vi "advent_2.vi"() -> ()   [LabVIEW 2021]
uses:
  <vilib>/Utility/file.llb/Read Delimited Spreadsheet (string).vi
panel:
  out "old depth equals aim":bool
  out "Horizontals equal?":bool
  out "Aim":i32
  out "horizontal * Depth 2":i32
  out "horizontal 2":i32
  out "Depth 2":i32
  out "min value":i32
  out "max value":i32
  out "size(s)":i32
  out "Depth":i32
  out "horizontal":i32
  out "horizontal * Depth":i32
  out "both same size":bool
  out "all rows":string[][](array[string])
  # "900"
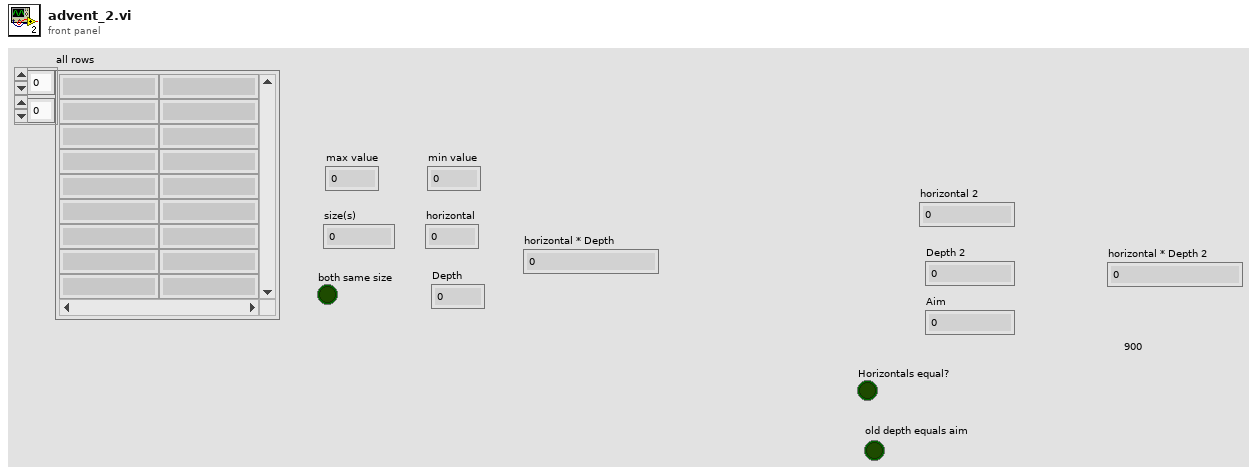
[diagram p1: front panel]
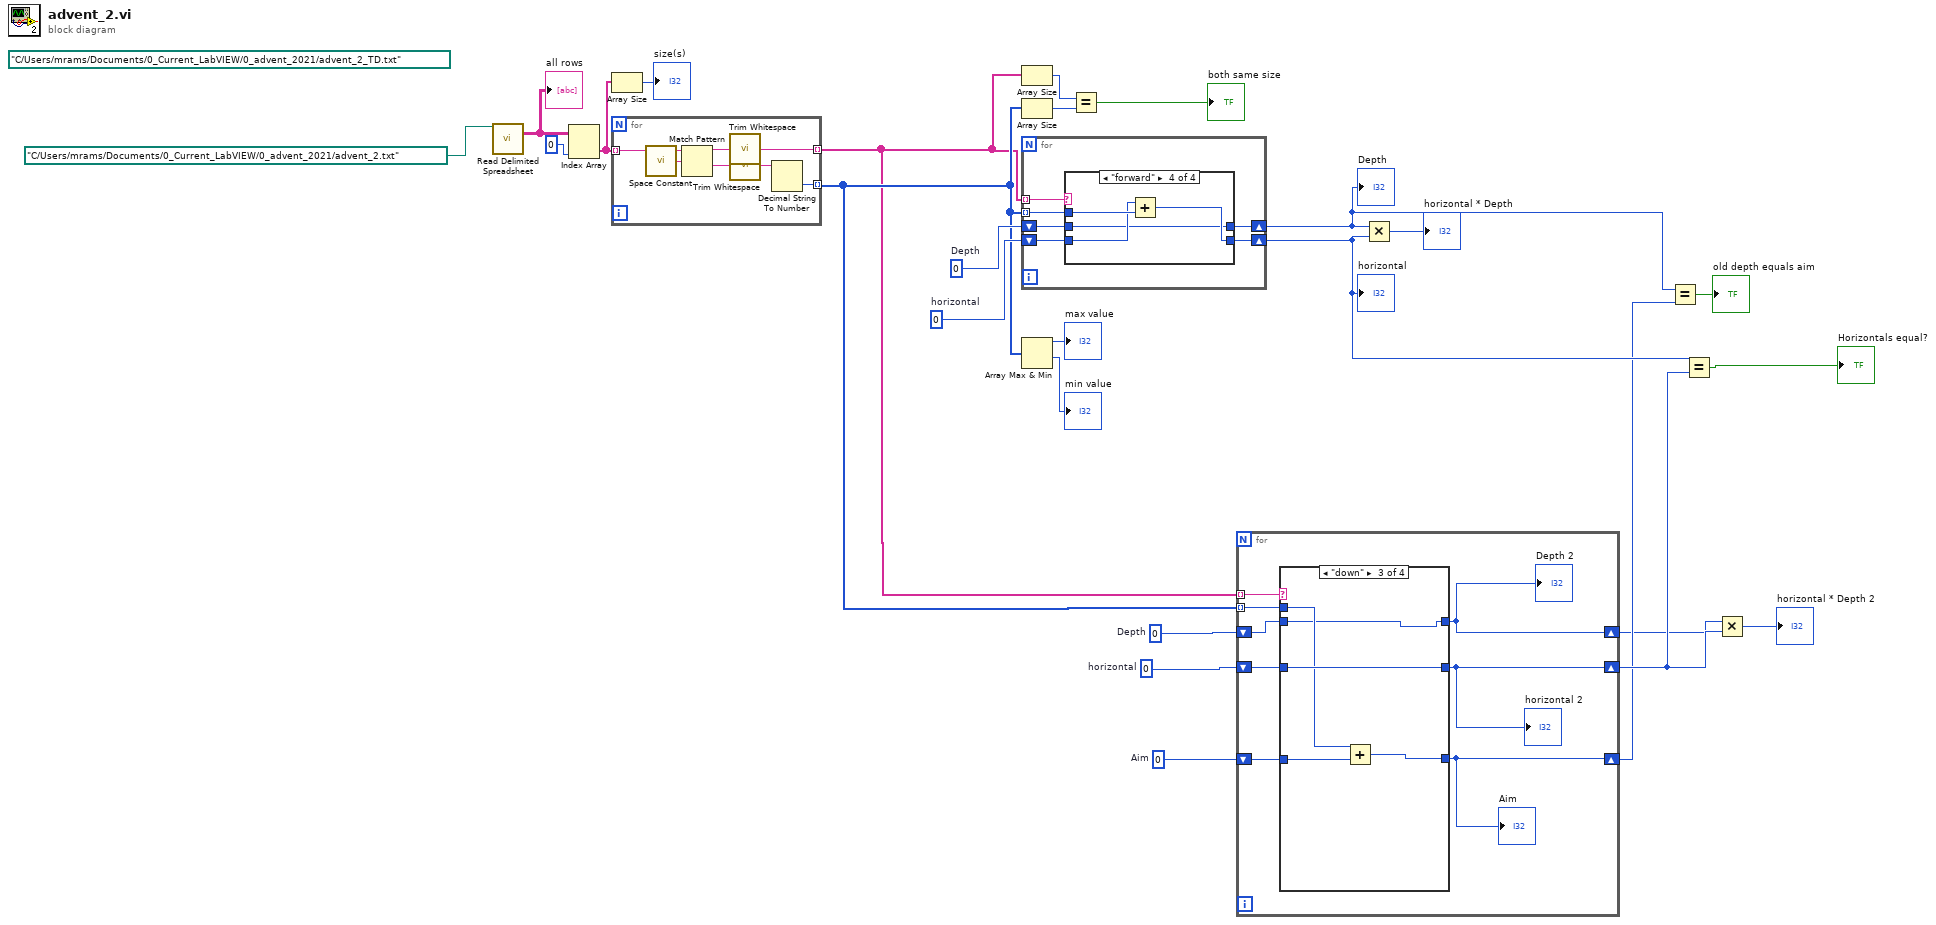
[diagram p0: block diagram]
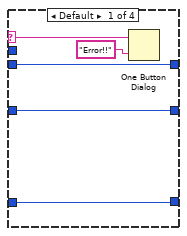
[diagram p2: hidden frame]
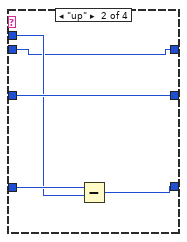
[diagram p3: hidden frame]
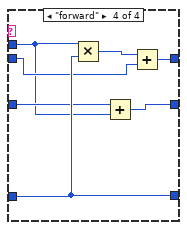
[diagram p4: hidden frame]
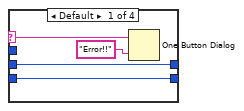
[diagram p5: hidden frame]
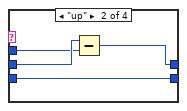
[diagram p6: hidden frame]
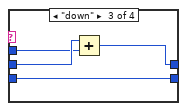
[diagram p7: hidden frame]
diagram:
  (unwired) path "C:/Users/mrams/Documents/0_Current_LabVIEW/0_advent_2021/advent_2_TD.txt" ("file path (dialog if empty)")
  w10 = 0  # Aim
  w12 = 0  # Depth
  w13 = 0  # horizontal
  w21 = 0  # Depth
  w20 = 0  # horizontal
  n1 = call-poly <vilib>:"Read Delimited Spreadsheet.vi"("file path (dialog if empty)"=path "C:/Users/mrams/Documents/0_Current_LabVIEW/0_advent_2021/advent_2.txt") -> ("all rows"=w25:string[][])  [unwired: 9 in, 5 out]
  "all rows" <- w25
  n2 = Index Array(array=w25, index (col)=0 ("disabled index (col)")) -> (element=w18:string[])  [unwired: 1 in]
  n3 = Array Size(array=w18) -> (size(s)=→"size(s)":i32)
  n4 = for {
    tunnel: w18 -> [w32] mode=indexing
    tunnel: [w28] -> w3 mode=indexing
    tunnel: [w29] -> w11 mode=indexing
    n5 = call <vilib>:"Space Constant.vi"() -> ("String"=w33:string)
    n6 = Match Pattern(string=w32, regular expression=w33) -> (before substring=w31:string, after substring=w30:string)  [unwired: 1 in, 2 out]
    n7 = call <vilib>:"Trim Whitespace.vi"("string"=w31) -> ("trimmed string"=w28:string)  [unwired: 1 in]
    n8 = call <vilib>:"Trim Whitespace.vi"("string"=w30) -> ("trimmed string"=w27:string)  [unwired: 1 in]
    n9 = Decimal String To Number(string=w27) -> (number=w29:i32)  [unwired: 2 in, 1 out]
  }
  n10 = Array Size(array=w3) -> (size(s)=w24:i32)
  n11 = Array Size(array=w11) -> (size(s)=w23:i32)
  n12 = for {
    tunnel: w3 -> [w39] mode=indexing
    tunnel: w11 -> [w37] mode=indexing
    shift-right: [w35] -> w5
    shift-left: w21 -> [w38]
    shift-right: [w34] -> w9
    shift-left: w20 -> [w36]
    n13 = case shown="\"forward\"" w39 {
      selector: w39 -> [w43 _ _ _]
      tunnel: w38 -> [w41 w47 w51 w52]
      tunnel: w37 -> [_ w46 w50 w55]
      tunnel: w36 -> [w40 w44 w48 w54]
      tunnel: [w41 w45 w49 w52] -> w35
      tunnel: [w40 w44 w48 w53] -> w34
      frame Default {
        n14 = One Button Dialog(message=w43, button name ("OK")="Error!!") -> ()  [unwired: 1 out]
      }
      frame "up" {
        n15 = Subtract(x=w47, y=w46) -> (x-y=w45:i32)
      }
      frame "down" {
        n16 = Add(x=w51, y=w50) -> (x+y=w49:i32)
      }
      frame "forward" {
        n17 = Add(x=w54, y=w55) -> (x+y=w53:i32)
      }
    }
  }
  "horizontal" <- w9
  "Depth" <- w5
  n18 = Array Max & Min(array=w11) -> (max value=→"max value":i32, min value=→"min value":i32)  [unwired: 2 out]
  n19 = Equal?(x=w24, y=w23) -> (x = y?=→"both same size":bool)
  n20 = for {
    tunnel: w3 -> [w63] mode=indexing
    tunnel: w11 -> [w61] mode=indexing
    shift-right: [w59] -> w2
    shift-left: w12 -> [w62]
    shift-right: [w58] -> w7
    shift-left: w13 -> [w60]
    shift-right: [w56] -> w6
    shift-left: w10 -> [w57]
    n21 = case shown="\"down\"" w63 {
      selector: w63 -> [w68 _ _ _]
      tunnel: w62 -> [w66 w69 w74 w80]
      tunnel: w61 -> [_ w70 w75 w79]
      tunnel: w60 -> [w65 w73 w78 w83]
      tunnel: [w66 w69 w74 w82] -> w59
      tunnel: [w65 w73 w78 w81] -> w58
      tunnel: w57 -> [w64 w72 w77 w84]
      tunnel: [w64 w71 w76 w84] -> w56
      frame Default {
        n22 = One Button Dialog(message=w68, button name ("OK")="Error!!") -> ()  [unwired: 1 out]
      }
      frame "up" {
        n23 = Subtract(x=w72, y=w70) -> (x-y=w71:i32)
      }
      frame "down" {
        n24 = Add(x=w75, y=w77) -> (x+y=w76:i32)
      }
      frame "forward" {
        n25 = Multiply(x=w79, y=w84) -> (x*y=w85:i32)
        n26 = Add(x=w83, y=w79) -> (x+y=w81:i32)
        n27 = Add(x=w85, y=w80) -> (x+y=w82:i32)
      }
    }
    "Depth 2" <- w59
    "Aim" <- w56
    "horizontal 2" <- w58
  }
  n28 = Multiply(x=w5, y=w9) -> (x*y=→"horizontal * Depth":i32)
  n29 = Equal?(x=w5, y=w6) -> (x = y?=→"old depth equals aim":bool)
  n30 = Equal?(x=w9, y=w7) -> (x = y?=→"Horizontals equal?":bool)
  n31 = Multiply(x=w2, y=w7) -> (x*y=→"horizontal * Depth 2":i32)
